vi "test Loopback_Acyclic_withOverflow.vi"(8 "error in":errorcluster, 11 "TestCase in":refnum<class "Single Core Acyclic Loopback.lvclass">) -> (0 "error out":errorcluster, 3 "TestCase out":refnum<class "Single Core Acyclic Loopback.lvclass">)   [LabVIEW 2020, in "Single Core Acyclic Loopback.lvclass"]
uses:
  Single Core Acyclic Loopback.lvclass
  C:/Git/niveristand-custom-device-testing-tools/VeriStandTestCase/VeriStandTestCase.lvclass
  <vilib>/numeric/Random Number (Range) I64.vi
  <vilib>/numeric/sub_Random U32.vi
  <vilib>/NI VeriStand/Execution/Workspace/NI VeriStand - Set Multiple Channel Values.vi
  <vilib>/NI VeriStand/Execution/Workspace/NI VeriStand - Set Single Channel Value.vi
  <vilib>/NI VeriStand/Execution/Workspace/NI VeriStand - Get Single Channel Value.vi
  <vilib>/addons/_JKI Toolkits/VI Tester/TestCase.llb/TestCase.lvclass
  <vilib>/NI VeriStand/Execution/Workspace/NI_VS Workspace ExecutionAPI.lvlib
  niveristand-custom-device-testing-tools/VeriStandTestUtilities/VeriStandTestUtilities.lvlib
  C:/Program Files (x86)/National Instruments/LabVIEW 2020/vi.lib/addons/_JKI Toolkits/VI Tester/TestCase.llb/TestCase.lvclass
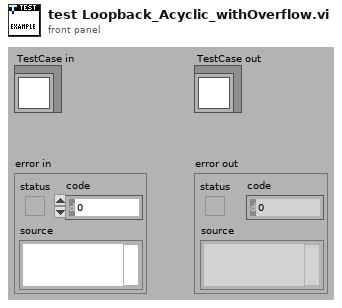
[diagram p1: front panel]
types:
  T1 = typedef "NI_VS Workspace ExecutionAPI.lvlib/WorkspaceAPI.ctl" = refnum<k24>
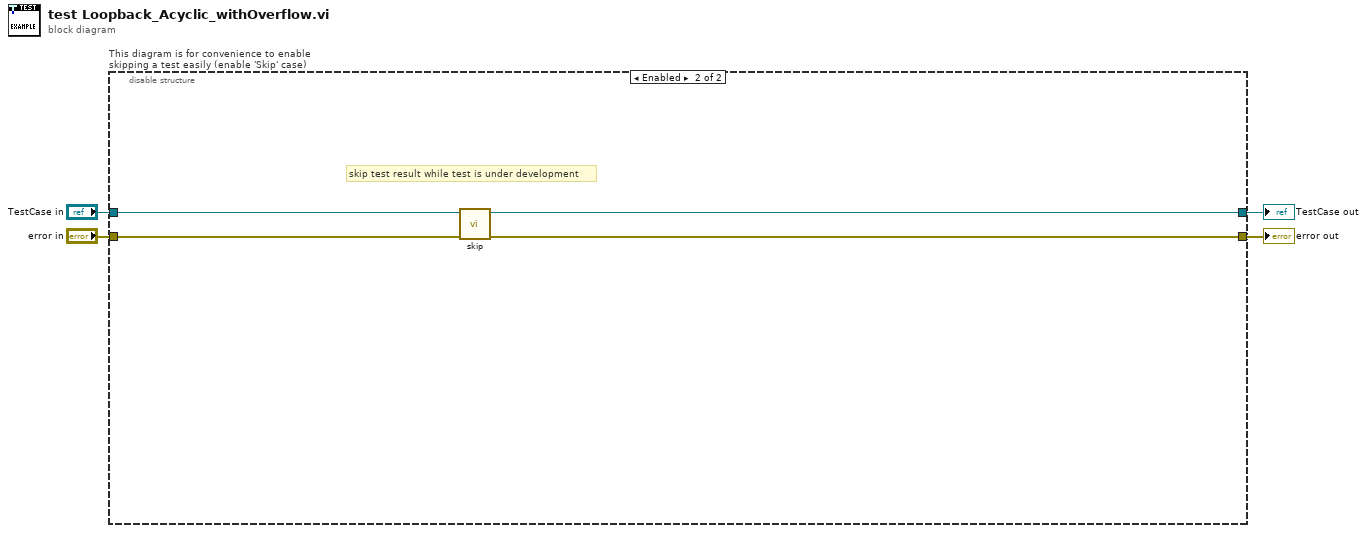
[diagram p0: block diagram]
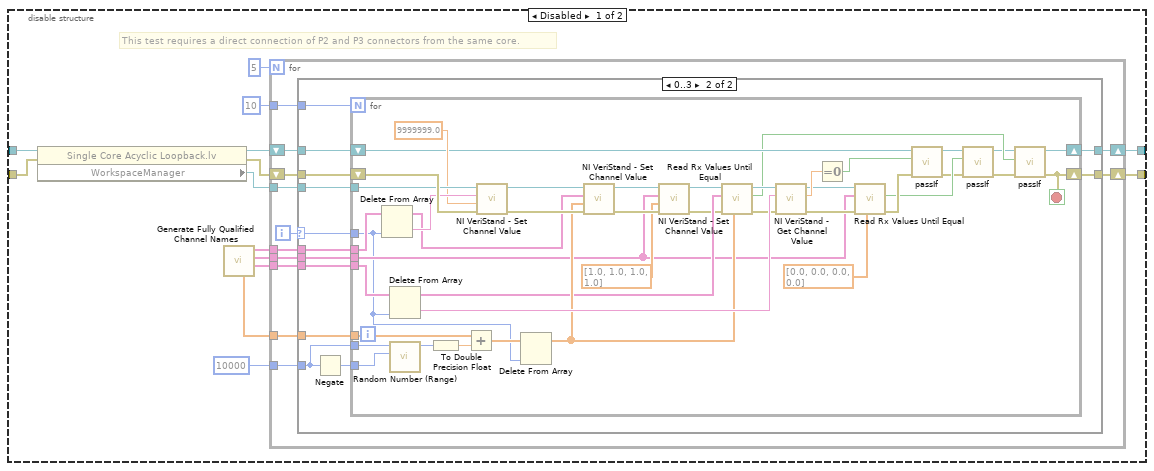
[diagram p2: hidden frame]
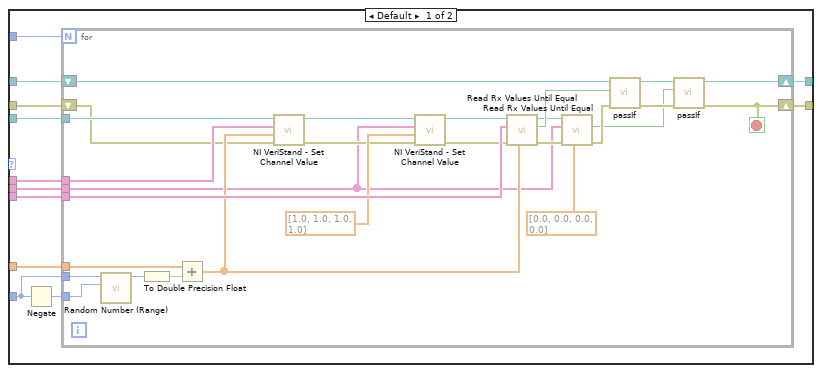
[diagram p3: hidden frame]
diagram:
  n1 = disable-structure "This diagram is for convenience to enable skipping a test easily (enable 'Skip' case)" shown="Enabled" {
    disable-tunnel: "TestCase in" -> [w18 w128]
    disable-tunnel: [w6 w126] -> w1
    disable-tunnel: [w5 w127] -> w3
    disable-tunnel: "error in" -> [w17 w125]
    frame Disabled {
      # "This test requires a direct connection of P2 and P3 connectors from the same core."
      n2 = property class="Single Core Acyclic Loopback.lv"(reference=w18, error in=w17) -> (reference out=w13:refnum<class "Single Core Acyclic Loopback.lvclass">, error out=w14:errorcluster, "WorkspaceManager"=w15:T1)
      n3 = call "Generate Fully Qualified Channel Names.vi"() -> ("Rx channels"=w8:string[], "trigger channels"=w9:string[], "Tx channels"=w10:string[], "channel index"=w7:dbl[])  [unwired: 8 in]
      n4 = for {
        N: 5 -> [_]
        tunnel: w7 -> [w30]
        tunnel: i64 10000 ("upper bound (100)") -> [w29]
        tunnel: w10 -> [w28]
        tunnel: w15 -> [w27]
        tunnel: w8 -> [w25]
        shift-right: [w22] -> w5
        shift-left: w14 -> [w26]
        shift-right: [w23] -> w6
        shift-left: w13 -> [w24]
        tunnel: w9 -> [w20]
        tunnel: 10 -> [w19]
        i -> [w21]
        n5 = case shown="0..3" w21 {
          selector: w21 -> [_ w72]
          tunnel: w30 -> [w42 w82]
          tunnel: w29 -> [w41 w81]
          tunnel: w28 -> [w39 w79]
          tunnel: w27 -> [w38 w78]
          tunnel: w26 -> [w37 w77]
          tunnel: w25 -> [w36 w76]
          tunnel: w24 -> [w35 w75]
          tunnel: [w34 w74] -> w23
          tunnel: [w33 w73] -> w22
          tunnel: w20 -> [w32 w71]
          tunnel: w19 -> [w31 w70]
          frame Default {
            n6 = Negate(x=w41) -> (-x=w40:i64)
            n7 = for {
              N: w31 -> [_]
              tunnel: w42 -> [w67]
              tunnel: w41 -> [w66]
              tunnel: w40 -> [w65]
              tunnel: w39 -> [w64]
              tunnel: w38 -> [w58]
              tunnel: w36 -> [w63]
              shift-right: [w49] -> w34
              shift-left: w35 -> [w62]
              shift-right: [w50] -> w33
              shift-left: w37 -> [w53]
              tunnel: w32 -> [w44]
              stop <- w50 stop-if-true
              n8 = call-poly <vilib>:"Random Number (Range).vi"("lower bound (-100)"=w65, "upper bound (100)"=w66) -> ("number"=w69:i64)  [unwired: 9 in]
              n9 = To Double Precision Float(number=w69) -> (double precision float=w68:dbl)
              n10 = Add(x=w67, y=w68) -> (x+y=w61:dbl[])
              n11 = call-poly <vilib>:"NI VeriStand - Set Channel Value.vi"("error in (no error)"=w53, "Values"=w61, "Channels"=w64, "WorkspaceManager in"=w58) -> ("error out"=w54:errorcluster, "WorkspaceManager out"=w57:T1)  [unwired: 6 in]
              n12 = call-poly <vilib>:"NI VeriStand - Set Channel Value.vi"("error in (no error)"=w54, "Values"=dbl[] [1.0, 1.0, 1.0, 1.0], "Channels"=w44, "WorkspaceManager in"=w57) -> ("error out"=w55:errorcluster, "WorkspaceManager out"=w56:T1)  [unwired: 6 in]
              n13 = call "Read Rx Values Until Equal.vi"("expected values"=w61, "error in"=w55, "Rx aliases"=w63, "workspace manager in"=w56) -> ("error out"=w48:errorcluster, "values equal expected"=w60:bool, "workspace manager out"=w47:T1)  [unwired: 5 in]
              n14 = call "Read Rx Values Until Equal.vi"("expected values"=dbl[] [0.0, 0.0, 0.0, 0.0] ("Values"), "error in"=w48, "Rx aliases"=w44, "workspace manager in"=w47) -> ("error out"=w46:errorcluster, "values equal expected"=w45:bool)  [unwired: 5 in, 1 out]
              n15 = call-dynamic "passIf.vi"("error in (no error)"=w46, "pass"=w60, "TestCase in"=w62) -> ("error out"=w51:errorcluster, "TestCase out"=w52:refnum<class "Single Core Acyclic Loopback.lvclass">)  [unwired: 7 in]
              n16 = call-dynamic "passIf.vi"("error in (no error)"=w51, "pass"=w45, "TestCase in"=w52) -> ("error out"=w50:errorcluster, "TestCase out"=w49:refnum<class "Single Core Acyclic Loopback.lvclass">)  [unwired: 7 in]
            }
          }
          frame 0..3 {
            n17 = Negate(x=w81) -> (-x=w80:i64)
            n18 = for {
              N: w70 -> [_]
              tunnel: w82 -> [w122]
              tunnel: w81 -> [w121]
              tunnel: w80 -> [w120]
              tunnel: w79 -> [w117]
              tunnel: w78 -> [w114]
              tunnel: w76 -> [w116]
              shift-right: [w119] -> w74
              shift-left: w75 -> [w109]
              shift-right: [w118] -> w73
              shift-left: w77 -> [w115]
              tunnel: w72 -> [w83]
              tunnel: w71 -> [w91]
              stop <- w118 stop-if-true
              n19 = Delete From Array(array=w117, index=w83) -> (deleted portion=w113:string, array with subset deleted=w84:string[])  [unwired: 1 in]
              n20 = Delete From Array(array=w116, index=w83) -> (deleted portion=w111:string, array with subset deleted=w100:string[])  [unwired: 1 in]
              n21 = call-poly <vilib>:"Random Number (Range).vi"("lower bound (-100)"=w120, "upper bound (100)"=w121) -> ("number"=w124:i64)  [unwired: 9 in]
              n22 = To Double Precision Float(number=w124) -> (double precision float=w123:dbl)
              n23 = Add(x=w122, y=w123) -> (x+y=w107:dbl[])
              n24 = call-poly <vilib>:"NI VeriStand - Set Channel Value.vi"("error in (no error)"=w115, "Value"=9999999.0, "Channel"=w113, "WorkspaceManager in"=w114) -> ("error out"=w103:errorcluster, "WorkspaceManager out"=w104:T1)  [unwired: 6 in]
              n25 = Delete From Array(array=w107, index=w83) -> (array with subset deleted=w101:dbl[])  [unwired: 1 in, 1 out]
              n26 = call-poly <vilib>:"NI VeriStand - Set Channel Value.vi"("error in (no error)"=w103, "Values"=w101, "Channels"=w84, "WorkspaceManager in"=w104) -> ("error out"=w105:errorcluster, "WorkspaceManager out"=w106:T1)  [unwired: 6 in]
              n27 = call-poly <vilib>:"NI VeriStand - Set Channel Value.vi"("error in (no error)"=w105, "Values"=dbl[] [1.0, 1.0, 1.0, 1.0], "Channels"=w91, "WorkspaceManager in"=w106) -> ("error out"=w98:errorcluster, "WorkspaceManager out"=w99:T1)  [unwired: 6 in]
              n28 = call "Read Rx Values Until Equal.vi"("expected values"=w101, "error in"=w98, "Rx aliases"=w100, "workspace manager in"=w99) -> ("error out"=w96:errorcluster, "values equal expected"=w95:bool, "workspace manager out"=w97:T1)  [unwired: 5 in]
              n29 = call-poly <vilib>:"NI VeriStand - Get Channel Value.vi"("error in (no error)"=w96, "Channel"=w111, "WorkspaceManager in"=w97) -> ("error out"=w94:errorcluster, "Value"=w110:dbl, "WorkspaceManager out"=w92:T1)  [unwired: 6 in]
              n30 = Equal To 0?(x=w110) -> (x = 0?=w108:bool)
              n31 = call "Read Rx Values Until Equal.vi"("expected values"=dbl[] [0.0, 0.0, 0.0, 0.0] ("Values"), "error in"=w94, "Rx aliases"=w91, "workspace manager in"=w92) -> ("error out"=w93:errorcluster, "values equal expected"=w89:bool)  [unwired: 5 in, 1 out]
              n32 = call-dynamic "passIf.vi"("error in (no error)"=w93, "pass"=w108, "TestCase in"=w109) -> ("error out"=w87:errorcluster, "TestCase out"=w88:refnum<class "Single Core Acyclic Loopback.lvclass">)  [unwired: 7 in]
              n33 = call-dynamic "passIf.vi"("error in (no error)"=w87, "pass"=w89, "TestCase in"=w88) -> ("error out"=w85:errorcluster, "TestCase out"=w86:refnum<class "Single Core Acyclic Loopback.lvclass">)  [unwired: 7 in]
              n34 = call-dynamic "passIf.vi"("error in (no error)"=w85, "pass"=w95, "TestCase in"=w86) -> ("error out"=w118:errorcluster, "TestCase out"=w119:refnum<class "Single Core Acyclic Loopback.lvclass">)  [unwired: 7 in]
            }
          }
        }
      }
    }
    frame Enabled {
      # "skip test result while test is under development"
      n35 = call <vilib>:"skip.vi"("error in (no error)"=w125, "TestCase in"=w128) -> ("error out"=w127:errorcluster, "TestCase out"=w126:refnum<class "Single Core Acyclic Loopback.lvclass">)  [unwired: 8 in]
    }
  }
  "error out" <- w3
  "TestCase out" <- w1
